vi "Read Storage Status.vi"(8 "error in (no error)":errorcluster, 10 "Read Req":T3, 11 "Device ID (0)":i32) -> (0 "error out":errorcluster, 2 "Storage Status Rsp":T2, 3 "Device ID out":i32, 4 "Storage Info":T1)   [LabVIEW 8.6, in "Keyence LJ-V7000.lvlib"]
doc: "fWhen the storage target setting is not off, this function gets the storage status."
uses:
  Keyence LJ-V7000.lvlib
  constant/Driver VI No.ctl
  Clusters/Read Storage Status Rsp.ctl
  Clusters/Storage Info.ctl
  Clusters/Read Storage Status Req.ctl
panel:
  # "(c) 2012 KEYENCE CORPORATION.  ALL RIGHTS RESERVED."
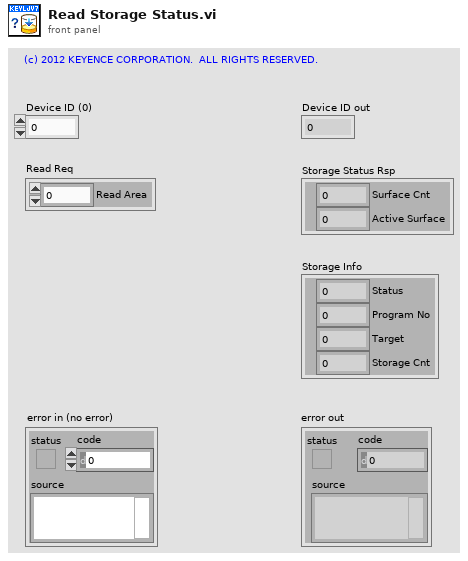
[diagram p1: front panel]
types:
  T1 = typedef "Keyence LJ-V7000.lvlib/Storage Info.ctl" = cluster{"Status":u8, "Program No":u8, "Target":u8, "Storage Cnt":u32}
  T2 = typedef "Keyence LJ-V7000.lvlib/Read Storage Status Rsp.ctl" = cluster{"Surface Cnt":u32, "Active Surface":u32}
  T3 = typedef "Keyence LJ-V7000.lvlib/Read Storage Status Req.ctl" = cluster{"Read Area":u32}
  T4 = typedef "Keyence LJ-V7000.lvlib/Driver VI No.ctl" = enum16{"Initialize", "Close", "Reboot Controller", "Return to Factory State", "Get System Error", "Clear System Error", "Trigger", "Start Batch Measurements", "Stop Batch Measurements", "Auto Zero", "Timing", "Reset", "Clear Memory", "Set Setting", "Get Setting", "Initialize Setting", "Reflect Setting", "Update Write Settings Area", "Check Status of Saving to Save Area", "Set Time", "Get Time", "Change Program", "Read Active Program Number", "Read Measurement Data", "Read Profiles(for High-Speed Mode)", "Read Batch Profiles(for High-Speed Mode)", "Read Profiles(for Advanced Mode)", "Read Batch Profiles(for Advanced Mode)", "Start Storage", "Stop Storage", "Read Storage Status", "Read Data Storage Data", "Read Profile Storage Data", "Read Batch Profile Storage Data", "Start High-Speed Data Communication", "Stop High-Speed Data Communication", "Read Profiles(for High-Speed Communication)"}
  T5 = cluster{"Status":u8, "Program No":u8, "Target":u8, "reserved":u8, "reserved":u8, "reserved":u8, "reserved":u8, "reserved":u8, "Storage Cnt":u32}
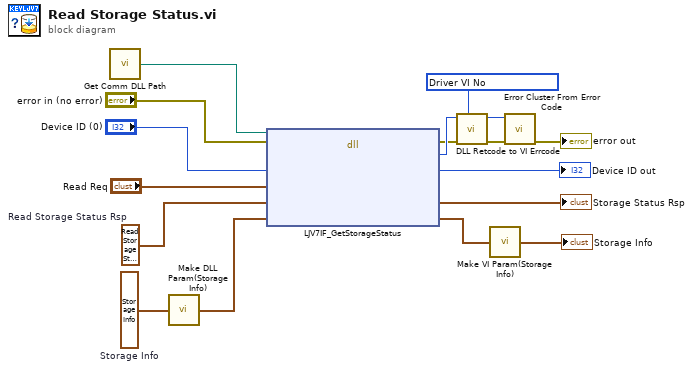
[diagram p0: block diagram]
diagram:
  w10 = T1 ?  # Storage Info
  w12 = T2 ?  # Read Storage Status Rsp
  n1 = call "Get Comm DLL Path.vi"() -> ("Comm DLL Path"=w15:path)  [unwired: 1 in]
  n2 = call "Make DLL Param(Storage Info).vi"("Storage Info"=w10) -> ("pStorageInfo"=w9:T5)
  n3 = dll-call lib="C:/Program Files/National Instruments/LabVIEW 2011/instr.lib/Keyence LJ-V7000/LJV7_IF.*" fn="LJV7IF_GetStorageStatus"(path in=w15, error in="error in (no error)", "lDeviceId"="Device ID (0)", "pReq"="Read Req", "pRsp"=w12, "pStorageInfo"=w9) -> (error out=w3:errorcluster, "lRetCode"=w4:i32, "lDeviceId"=→"Device ID out":i32, "pRsp"=→"Storage Status Rsp":T2, "pStorageInfo"=w7:T5)  [unwired: 2 in, 1 out]
  n4 = call "DLL Retcode to VI Errcode.vi"("Driver VI No"=T4 ?, "error in (no error)"=w3, "DLL Return Code"=w4) -> ("error out"=w6:errorcluster, "VI Error Code"=w5:i32)  [unwired: 7 in]
  n5 = call "Make VI Param(Storage Info).vi"("pStorageInfo"=w7) -> ("Storage Info"=→"Storage Info":T1)
  n6 = call <vilib>:"Error Cluster From Error Code.vi"("error in (no error)"=w6, "error code (0)"=w5) -> ("error out"=→"error out":errorcluster)  [unwired: 7 in]
